vi "GenerateApriltag16h5.vi"(8 "error in (no error)":errorcluster, 11 "ID":i32) -> (0 "error out":errorcluster, 3 "Tag Pixel Array":u8[][](array[numeric]) format="%.0x")   [LabVIEW 2020, in "feature_detection.lvlib"]
uses:
  feature_detection.lvlib
  TagIDOutOfRangeError.vi
  <vilib>/Utility/error.llb/Error Cluster From Error Code.vi
  TagLayoutConvert.vi
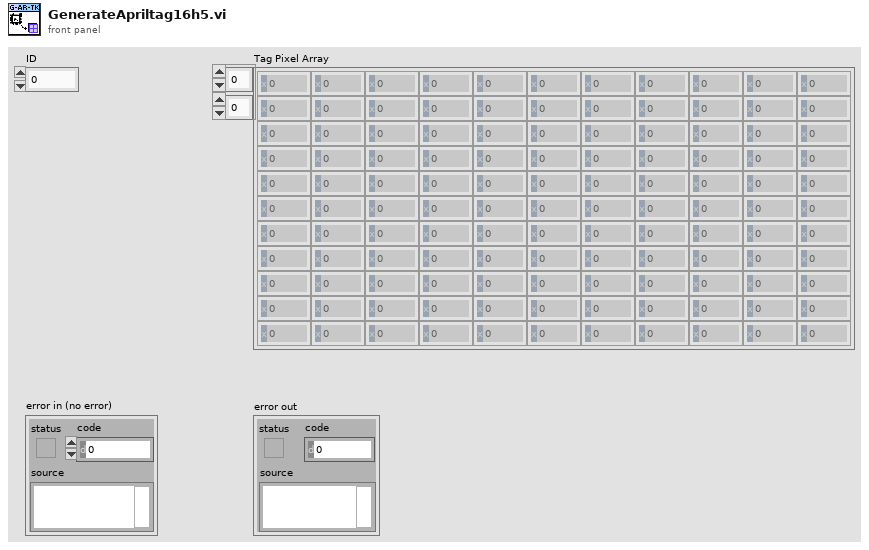
[diagram p1: front panel]
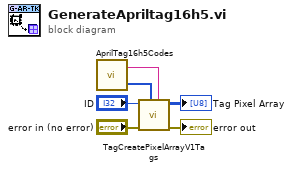
[diagram p0: block diagram]
diagram:
  n1 = call "AprilTag16h5Codes.vi"() -> ("Codes"=w2:i64[], "Layout"=w3:string)  [unwired: 2 in]
  n2 = call "TagCreatePixelArrayV1Tags.vi"("Layout"=w3, "Codes"=w2, "error in (no error)"="error in (no error)", "ID"="ID") -> ("error out"=→"error out":errorcluster, "Pixels"=→"Tag Pixel Array":u8[][])  [unwired: 6 in]
